vi "Configure Load to Single Point-Single.vi"(8 "error in":errorcluster, 10 "measurement configuration":T1 {"Measurement timeout" format="%.3p"; "Load device voltage/current rating" format="%#_6pA"; "Load output function" items=["DC Voltage"=1006, "DC Current"=1007, "Pulse Voltage"=1049, "Pulse Current"=1050]; "Power ON/Source output function" items=["DC Voltage"=1006, "DC Current"=1007, "Pulse Voltage"=1049, "Pulse Current"=1050]; "Load sense" items=["Local"=1008, "Remote"=1009]; "Load transient response" items=["Slow"=1041, "Normal"=1038, "Fast"=1039, "Custom"=1042]; "Power ON/Source sense" items=["Local"=1008, "Remote"=1009]; "Source transient response" items=["Slow"=1041, "Normal"=1038, "Fast"=1039, "Custom"=1042]; "Measurement duration" format="%.3p"; "Aperture time" format="%.3p"; "Load current/voltage limit high" format="%#_6p"; "Load current/voltage limit low" format="%#_6p"; "Load current/voltage limit range" format="%#_6p"; "Load voltage/current level range" format="%#_6p"; "Load voltage/current level" format="%#_6p"; "Source current/voltage limit high" format="%#_6p"; "Source current/voltage limit low" format="%#_6p"; "Power ON/Source current/voltage limit range" format="%#_6p"; "Source voltage/current level range" format="%#_6p"; "Power ON/Source voltage/current level" format="%#_6p"}, 11 "Single Point Perform Measurement in":T2) -> (0 "error out":errorcluster, 3 "Single Point Perform Measurement out":T2)   [LabVIEW 2021, in "Single Point_Channel Ganging.lvlib"]
uses:
  Controls/Perform measurement-control.ctl
  shared subVIs/ctl/NIDCPower_channel_ganging - ctl - ganged session.ctl
  shared subVIs/ctl/NIDCPower_channel_ganging - ctl - ganged config.ctl
  shared subVIs/ctl/NIDCPower_channel_ganging - ctl - channel mode.ctl
  Measurement Results.ctl
  Measurement Configuration.ctl
  <instrlib>/niDCPower/nidcpower.llb/niDCPower Source Mode.ctl
  <instrlib>/niDCPower/nidcpower.llb/niDCPower Get Channel Name From String.vi
  Single Point_Channel Ganging.lvlib
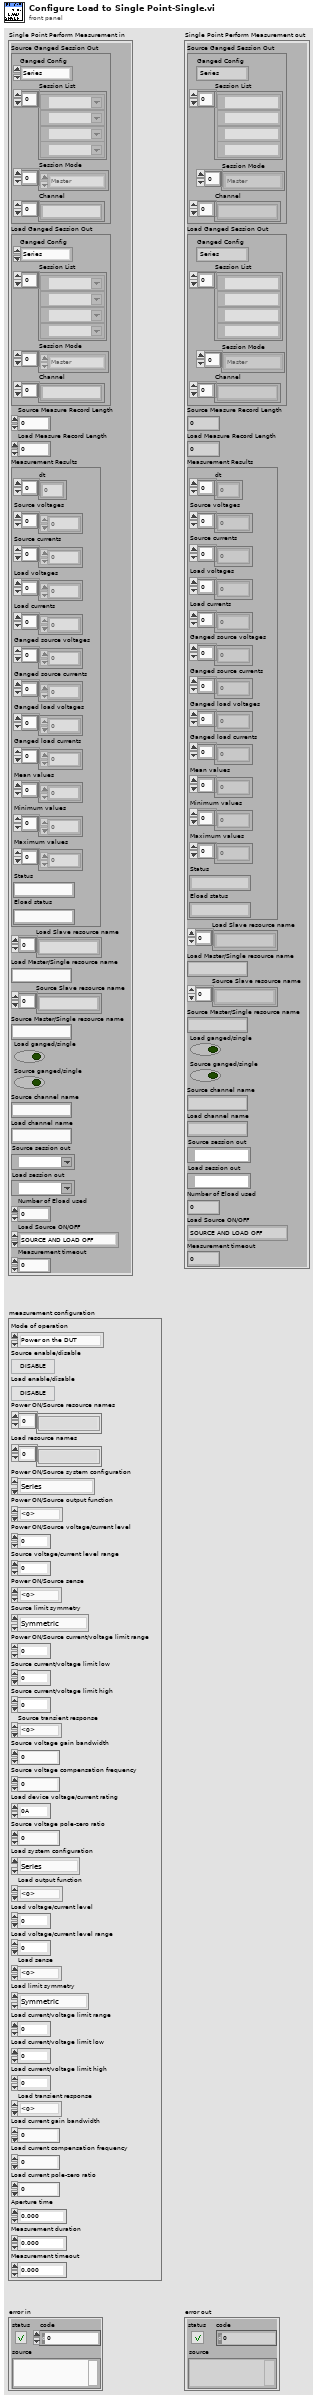
[diagram p1: front panel]
types:
  T1 = typedef "Single Point_Channel Ganging.lvlib/Measurement Configuration.ctl" = cluster{"Mode of operation":enum32{"Power on the DUT", "Perform measurement", "Power off the DUT"}, "Source enable/disable":bool, "Load enable/disable":bool, "Power ON/Source resource names":string[], "Load resource names":string[], "Power ON/Source system configuration":enum32{"Series", "Parallel", "Manual"}, "Power ON/Source output function":i32, "Power ON/Source voltage/current level":dbl, "Source voltage/current level range":dbl, "Power ON/Source sense":i32, "Source limit symmetry":enum32{"Symmetric", "Asymmetric"}, "Power ON/Source current/voltage limit range":dbl, "Source current/voltage limit low":dbl, "Source current/voltage limit high":dbl, "Source transient response":i32, "Source voltage gain bandwidth":dbl, "Source voltage compensation frequency":dbl, "Load device voltage/current rating":dbl, "Source voltage pole-zero ratio":dbl, "Load system configuration":enum32{"Series", "Parallel", "Manual"}, "Load output function":i32, "Load voltage/current level":dbl, "Load voltage/current level range":dbl, "Load sense":i32, "Load limit symmetry":enum32{"Symmetric", "Asymmetric"}, "Load current/voltage limit range":dbl, "Load current/voltage limit low":dbl, "Load current/voltage limit high":dbl, "Load transient response":i32, "Load current gain bandwidth":dbl, "Load current compensation frequency":dbl, "Load current pole-zero ratio":dbl, "Aperture time":dbl, "Measurement duration":dbl, "Measurement timeout":dbl}
  T2 = typedef "Single Point_Channel Ganging.lvlib/Perform measurement-control.ctl" = cluster{"Source Ganged Session Out":T3, "Load Ganged Session Out":T3, "Source Measure Record Length":i32, "Load Measure Record Length":i32, "Measurement Results":T6, "Load Slave resource name":string[], "Load Master/Single resource name":string, "Source Slave resource name":string[], "Source Master/Single resource name":string, "Load ganged/single":bool, "Source ganged/single":bool, "Source channel name":string, "Load channel name":string, "Source session out":refnum<k15>, "Load session out":refnum<k15>, "Number of Eload used":i32, "Load Source ON/OFF":enum16{"SOURCE AND LOAD OFF", "SOURCE ON", "LOAD ON", "SOURCE AND LAOD ON"}, "Measurement timeout":dbl}
  T3 = typedef "NIDCPower_channel_ganging - ctl - ganged session.ctl" = cluster{"Ganged Config":T4, "Session List":refnum<k15>[], "Session Mode":T5[], "Channel":string[]}
  T4 = typedef "NIDCPower_channel_ganging - ctl - ganged config.ctl" = enum32{"Series", "Parallel", "Manual"}
  T5 = typedef "NIDCPower_channel_ganging - ctl - channel mode.ctl" = enum32{"Master", "Slave", "Slave - Inverted"}
  T6 = typedef "Single Point_Channel Ganging.lvlib/Measurement Results.ctl" = cluster{"dt":dbl[], "Source voltages":dbl[], "Source currents":dbl[], "Load voltages":dbl[], "Load currents":dbl[], "Ganged source voltages":dbl[], "Ganged source currents":dbl[], "Ganged load voltages":dbl[], "Ganged load currents":dbl[], "Mean values":dbl[], "Minimum values":dbl[], "Maximum values":dbl[], "Status":string, "Eload status":string}
  T7 = typedef "niDCPower Source Mode.ctl" = i32
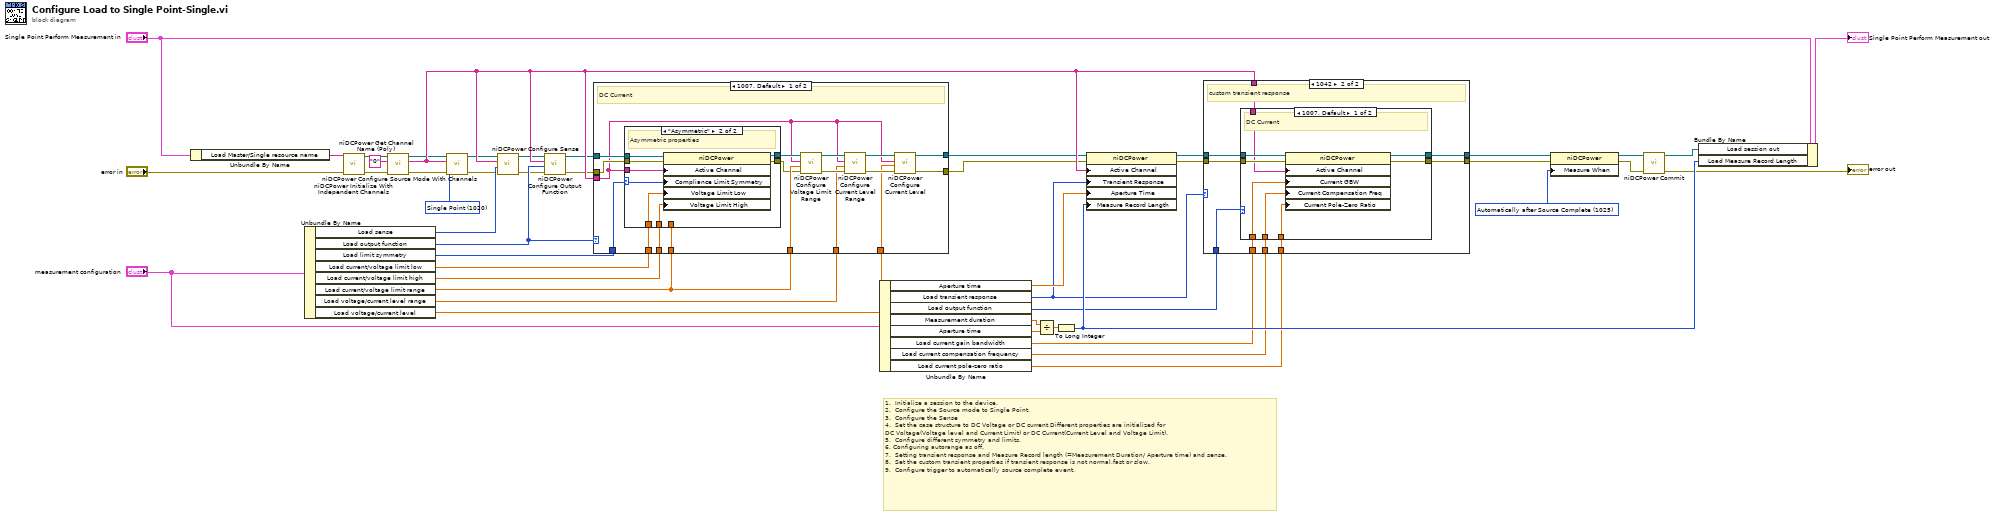
[diagram p0: block diagram]
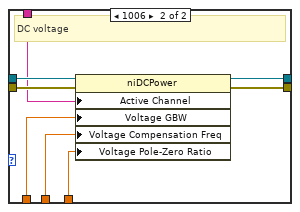
[diagram p3: hidden frame]
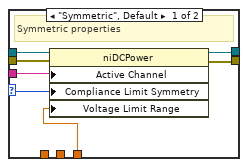
[diagram p4: hidden frame]
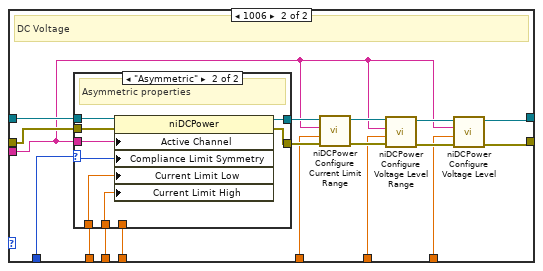
[diagram p5: hidden frame]
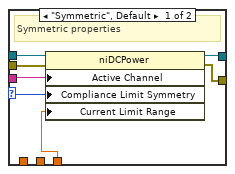
[diagram p6: hidden frame]
diagram:
  w32 = 1025 items=["Automatically after Source Complete"=1025, "On Demand"=1026, "On Measure Trigger"=1027] ("Measurement:Advanced:Measure When")
  w6 = T7 1020 items=["Single Point"=1020, "Sequence"=1021] ("source mode")
  # "1.  Initialize a session to the device.\n2.  Configure the Source mode to Single Point.\n3.  Configure the Sense\n4.  Set the case structure to DC Voltage or DC current.Different properties are initialized for \nDC Voltage(Voltage level and Current Limit) or DC Current(Current Level and Voltage Limit). \n5.  Configure different symmetry and limits.\n6. Configuring autorange as off.\n7.  Setting transient response and Measure Record length (=Measurement Duration/ Aperture time) and sense.\n8.  Set the custom transient properties if transient response is not normal,fast or slow.\n9.  Configure trigger to automatically source complete event."
  n1 = Unbundle By Name("Single Point Perform Measurement in") -> ("Load Master/Single resource name"=w20:string)
  n2 = Unbundle By Name("measurement configuration") -> ("Load sense"=w40:i32, "Load output function"=w41:i32, "Load limit symmetry"=w22:enum32{"Symmetric", "Asymmetric"}, "Load current/voltage limit low"=w23:dbl, "Load current/voltage limit high"=w24:dbl, "Load current/voltage limit range"=w25:dbl, "Load voltage/current level range"=w26:dbl, "Load voltage/current level"=w27:dbl)
  n3 = call <instrlib>:"niDCPower Initialize With Independent Channels.vi"("error in (no error)"="error in", "resource name"=w20) -> ("error out"=w3:errorcluster, "instrument handle out"=w1:refnum<k15>)  [unwired: 8 in]
  n4 = call-poly <instrlib>:"niDCPower Get Channel Name (Poly).vi"("error in (no error)"=w3, "index"="0", "instrument handle"=w1) -> ("error out"=w4:errorcluster, "name"=w21:string, "instrument handle out"=w5:refnum<k15>)  [unwired: 6 in]
  n5 = call <instrlib>:"niDCPower Configure Source Mode With Channels.vi"("error in (no error)"=w4, "source mode"=w6, "channel name"=w21, "instrument handle"=w5) -> ("error out"=w7:errorcluster, "instrument handle out"=w8:refnum<k15>)  [unwired: 6 in]
  n6 = call <instrlib>:"niDCPower Configure Sense.vi"("error in (no error)"=w7, "sense"=w40, "channel name"=w21, "instrument handle"=w8) -> ("error out"=w9:errorcluster, "instrument handle out"=w10:refnum<k15>)  [unwired: 6 in]
  n7 = call <instrlib>:"niDCPower Configure Output Function.vi"("error in (no error)"=w9, "output function"=w41, "channel name"=w21, "instrument handle"=w10) -> ("error out"=w12:errorcluster, "instrument handle out"=w11:refnum<k15>)  [unwired: 6 in]
  n8 = case shown="1007, Default" w41 {
    tunnel: w11 -> [w65 w98]
    tunnel: w12 -> [w64 w97]
    tunnel: w21 -> [w50 w83]
    tunnel: w22 -> [w49 w82]
    tunnel: w23 -> [w63 w96]
    tunnel: w24 -> [w62 w95]
    tunnel: w25 -> [w60 w88]
    tunnel: w26 -> [w56 w87]
    tunnel: w27 -> [w53 w86]
    tunnel: [w52 w85] -> w13
    tunnel: [w51 w84] -> w14
    tunnel: w25 -> [w48 w81]
    frame 1007, Default {
      # "DC Current"
      n9 = case shown="\"Asymmetric\"" w49 {
        selector: w49 -> [w72 w73]
        tunnel: w65 -> [w71 w80]
        tunnel: w64 -> [w70 w79]
        tunnel: w63 -> [_ w78]
        tunnel: w62 -> [_ w77]
        tunnel: [w68 w76] -> w61
        tunnel: [w67 w75] -> w59
        tunnel: w50 -> [w69 w74]
        tunnel: w48 -> [w66 _]
        frame "Symmetric", Default {
          # "Symmetric properties"
          n10 = property class="niDCPower"(reference=w71, error in=w70, "Active Channel"=w69, "Compliance Limit Symmetry"=w72, "Voltage Limit Range"=w66) -> (reference out=w68:refnum<k15>, error out=w67:errorcluster)
        }
        frame "Asymmetric" {
          # "Asymmetric properties"
          n11 = property class="niDCPower"(reference=w80, error in=w79, "Active Channel"=w74, "Compliance Limit Symmetry"=w73, "Voltage Limit Low"=w78, "Voltage Limit High"=w77) -> (reference out=w76:refnum<k15>, error out=w75:errorcluster)
        }
      }
      n12 = call <instrlib>:"niDCPower Configure Voltage Limit Range.vi"("error in (no error)"=w59, "voltage limit range"=w60, "channel name"=w50, "instrument handle"=w61) -> ("error out"=w58:errorcluster, "instrument handle out"=w57:refnum<k15>)  [unwired: 6 in]
      n13 = call <instrlib>:"niDCPower Configure Current Level Range.vi"("error in (no error)"=w58, "current level range"=w56, "channel name"=w50, "instrument handle"=w57) -> ("error out"=w55:errorcluster, "instrument handle out"=w54:refnum<k15>)  [unwired: 6 in]
      n14 = call <instrlib>:"niDCPower Configure Current Level.vi"("error in (no error)"=w55, "current level"=w53, "channel name"=w50, "instrument handle"=w54) -> ("error out"=w51:errorcluster, "instrument handle out"=w52:refnum<k15>)  [unwired: 6 in]
    }
    frame 1006 {
      # "DC Voltage"
      n15 = case shown="\"Asymmetric\"" w82 {
        selector: w82 -> [w102 w106]
        tunnel: w98 -> [w105 w113]
        tunnel: w97 -> [w104 w112]
        tunnel: w96 -> [_ w111]
        tunnel: w95 -> [_ w110]
        tunnel: [w99 w109] -> w94
        tunnel: [w100 w108] -> w93
        tunnel: w83 -> [w103 w107]
        tunnel: w81 -> [w101 _]
        frame "Symmetric", Default {
          # "Symmetric properties"
          n16 = property class="niDCPower"(reference=w105, error in=w104, "Active Channel"=w103, "Compliance Limit Symmetry"=w102, "Current Limit Range"=w101) -> (reference out=w100:refnum<k15>, error out=w99:errorcluster)
        }
        frame "Asymmetric" {
          # "Asymmetric properties"
          n17 = property class="niDCPower"(reference=w113, error in=w112, "Active Channel"=w107, "Compliance Limit Symmetry"=w106, "Current Limit Low"=w111, "Current Limit High"=w110) -> (reference out=w108:refnum<k15>, error out=w109:errorcluster)
        }
      }
      n18 = call <instrlib>:"niDCPower Configure Current Limit Range.vi"("error in (no error)"=w94, "current limit range"=w88, "channel name"=w83, "instrument handle"=w93) -> ("error out"=w92:errorcluster, "instrument handle out"=w91:refnum<k15>)  [unwired: 6 in]
      n19 = call <instrlib>:"niDCPower Configure Voltage Level Range.vi"("error in (no error)"=w92, "voltage level range"=w87, "channel name"=w83, "instrument handle"=w91) -> ("error out"=w90:errorcluster, "instrument handle out"=w89:refnum<k15>)  [unwired: 6 in]
      n20 = call <instrlib>:"niDCPower Configure Voltage Level.vi"("error in (no error)"=w90, "voltage level"=w86, "channel name"=w83, "instrument handle"=w89) -> ("error out"=w84:errorcluster, "instrument handle out"=w85:refnum<k15>)  [unwired: 6 in]
    }
  }
  n21 = Unbundle By Name("measurement configuration") -> ("Aperture time"=w44:dbl, "Load transient response"=w42:i32, "Load output function"=w43:i32, "Measurement duration"=w45:dbl, "Aperture time"=w46:dbl, "Load current gain bandwidth"=w17:dbl, "Load current compensation frequency"=w18:dbl, "Load current pole-zero ratio"=w19:dbl)
  n22 = Divide(x=w45, y=w46) -> (x/y=w34:dbl)
  n23 = To Long Integer(number=w34) -> (32bit integer=w47:i32)
  n24 = property class="niDCPower"(reference=w13, error in=w14, "Active Channel"=w21, "Transient Response"=w42, "Aperture Time"=w44, "Measure Record Length"=w47) -> (reference out=w15:refnum<k15>, error out=w16:errorcluster)
  n25 = case shown="1042" w42 {
    tunnel: w43 -> [_ w124]
    tunnel: w15 -> [w114 w123]
    tunnel: w16 -> [w115 w122]
    tunnel: w17 -> [_ w121]
    tunnel: w18 -> [_ w120]
    tunnel: w19 -> [_ w119]
    tunnel: w21 -> [_ w118]
    tunnel: [w114 w117] -> w30
    tunnel: [w115 w116] -> w31
    frame Default {
      # "Normal, fast and slow transient"
    }
    frame 1042 {
      # "custom transient response"
      n26 = case shown="1007, Default" w124 {
        tunnel: w123 -> [w132 w140]
        tunnel: w122 -> [w131 w139]
        tunnel: w121 -> [w130 w138]
        tunnel: w120 -> [w129 w137]
        tunnel: w119 -> [w128 w136]
        tunnel: w118 -> [w127 w135]
        tunnel: [w126 w134] -> w117
        tunnel: [w125 w133] -> w116
        frame 1007, Default {
          # "DC Current"
          n27 = property class="niDCPower"(reference=w132, error in=w131, "Active Channel"=w127, "Current GBW"=w130, "Current Compensation Freq"=w129, "Current Pole-Zero Ratio"=w128) -> (reference out=w126:refnum<k15>, error out=w125:errorcluster)
        }
        frame 1006 {
          # "DC voltage"
          n28 = property class="niDCPower"(reference=w140, error in=w139, "Active Channel"=w135, "Voltage GBW"=w138, "Voltage Compensation Freq"=w137, "Voltage Pole-Zero Ratio"=w136) -> (reference out=w134:refnum<k15>, error out=w133:errorcluster)
        }
      }
    }
  }
  n29 = property class="niDCPower"(reference=w30, error in=w31, "Measure When"=w32) -> (reference out=w28:refnum<k15>, error out=w29:errorcluster)
  n30 = call <instrlib>:"niDCPower Commit.vi"("error in (no error)"=w29, "instrument handle"=w28) -> ("error out"=→"error out":errorcluster, "instrument handle out"=w33:refnum<k15>)  [unwired: 8 in]
  n31 = Bundle By Name(cluster="Single Point Perform Measurement in", "Load session out"=w33, "Load Measure Record Length"=w47) -> (→"Single Point Perform Measurement out":T2)
